vi "RF Rec Rx Streaming (Host).vi"() -> ()   [LabVIEW 2018]
doc: "This template is for the Simple NI-USRP Streaming design, a design that shows the basics of streaming data to and from an NI USRP-294x/295x device. Refer to the block diagram for more information about how to use this template."
uses:
  <vilib>/userdefined/Silver/nirio_resource_slv.ctl
  SubVIs/RF Rec Start Trigger.ctl
  <vilib>/Utility/error.llb/DialogType.ctl
panel:
  in  "config tab":enum32{"Rx Configuration"}(tab)
  in  "rx config":T2={"rf enable 0"=TRUE, "rf config 0"={"antenna"="RX2", "frequency"=2000000000.0, "lo frequency"=-1.0, "level"=0.0}, "rf enable 1"=TRUE, "rf config 1"={"antenna"="RX2", "frequency"=2000000000.0, "lo frequency"=-1.0, "level"=0.0}, "transfer mode"=enum."Finite", "sample rate"=10000000.0, "number of samples"=8192, "start trigger"=enum."Immediate"} {"sample rate" format="%#.3pS/s"; "rf config 1"."level" format="%#_gdBm"; "rf config 1"."lo frequency" format="%#.3pHz"; "rf config 1"."frequency" format="%#.3pHz"; "rf config 0"."level" format="%#_gdBm"; "rf config 0"."lo frequency" format="%#.3pHz"; "rf config 0"."frequency" format="%#.3pHz"}
  out "acquiring":bool caption="Acquiring"
  in  "USRP RIO device":T3="RIO0" caption="USRP RIO Device"
  in  "reference frequency source":string(combo)="Internal" caption="Reference Frequency Source"
  in  "indicator tab":T4(tab)
  out "power spectrum":cluster{"f0":dbl, "df":dbl, "magnitude":dbl[]}[](graph) caption="Power Spectrum"
  out "power level":dbl[][](graph) caption="Power Level"
  out "iq data":waveform(dbl)[](graph) caption="I & Q Data"
  out "rx.coerced config":T5 caption="Rx" {"coerced sample rates" format="%#.3pS/s"; "coerced levels" format="%#.3gdBm"; "coerced lo frequencies" format="%#.3pHz"; "coerced frequencies" format="%#.3pHz"}
  in  "rx.stop":bool
  # "This template is for the Simple NI-USRP Streaming design, a design that shows the basics of streaming data on a USRP RIO device. See the block diagram for more information on how to use this template."
  # "Simple Rx Streaming"
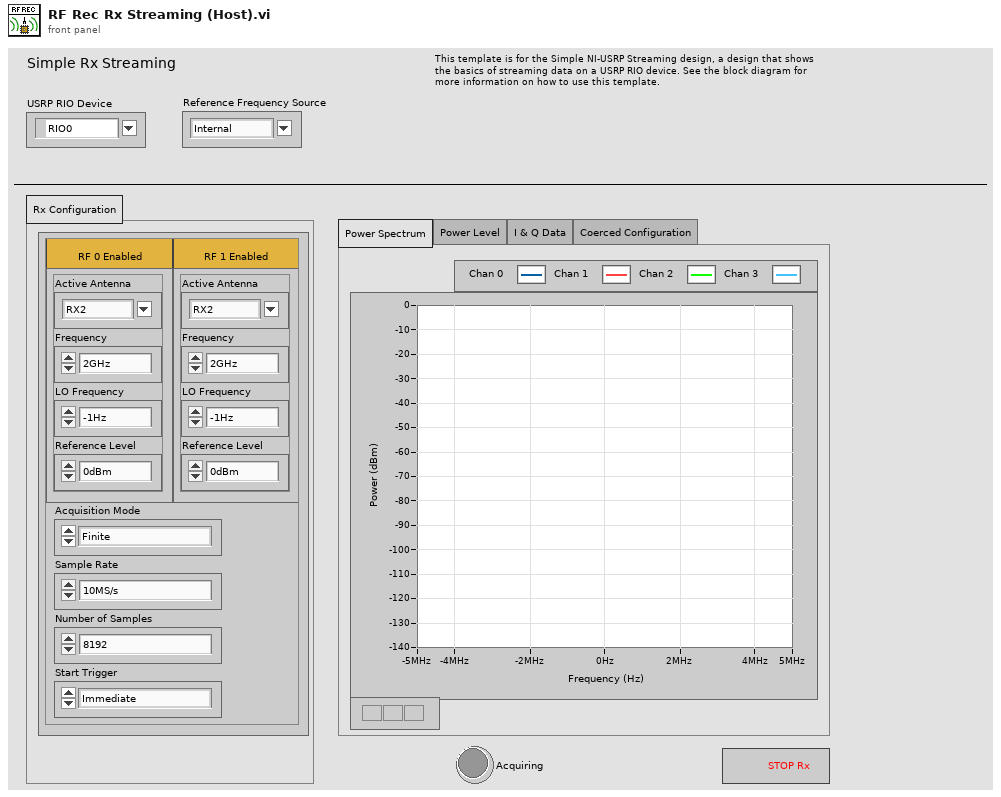
[diagram p1: front panel]
types:
  T1 = typedef "RF Rec Start Trigger.ctl" = enum8{"Software", "Digital Edge", "Rx Start Trigger", "Tx Start Trigger", "Immediate", "Future Time Event"}
  T2 = cluster{"rf enable 0":bool, "rf config 0":cluster{"antenna":string, "frequency":dbl, "lo frequency":dbl, "level":dbl}, "rf enable 1":bool, "rf config 1":cluster{"antenna":string, "frequency":dbl, "lo frequency":dbl, "level":dbl}, "transfer mode":enum16{"Finite", "Continuous"}, "sample rate":dbl, "number of samples":u32, "start trigger":T1}
  T3 = typedef "nirio_resource_slv.ctl" = tag
  T4 = enum32{"Power Spectrum", "Power Level", "I & Q Data", "Coerced Configuration"}
  T5 = cluster{"coerced frequencies":dbl[], "coerced lo frequencies":dbl[], "coerced levels":dbl[], "coerced sample rates":dbl[]}
  T6 = typedef "DialogType.ctl" = u16
  T7 = typedef "RF Rec Rx Channels.ctl" = cluster{"rx config":cluster{"channel configuration":cluster{"channel enable":bool, "channel configuration":cluster{"antenna":string, "frequency":dbl, "lo frequency":dbl, "level":dbl}}[], "transfer mode":enum16{"Finite", "Continuous"}, "sample rate":dbl, "number of samples":u32, "start trigger":T1}, "reference frequency source":string, "rx.data sink":enum16{"SFP Port 0", "SFP Port 1", "Host"}, "rx.enabled channels":string[], "vertical range":dbl[], "rx.coerced configurations":cluster{"coerced frequencies":dbl[], "coerced lo frequencies":dbl[], "coerced levels":dbl[], "coerced sample rates":dbl[]}}
  T8 = typedef "niUsrpRio Config v1 Host.lvlib/niUsrpRio Session.ctl" = cluster{"FPGA Interface":refnum<k20>, "RIO Interface Number":u32, "Data Clock Rate":u32, "FPGA Data Clock Rate":u32, "Global Settings Register Bus":T9, "Radio 0 Settings Register Bus":T9, "Radio 1 Settings Register Bus":T9, "Radio Settings Bus Semaphore":T10, "DB Queues":T11[], "Characterization Data Valid?":bool, "EEPROM Header":T12, "Device Data Header":T13, "EEPROM Characterization Header":T14, "Characterization Data":T15[], "FPGA Current Version":u32, "FPGA Oldest Compatible Version":u32, "Fixed Logic Current Version":u32, "Fixed Logic Oldest Compatible Version":u32, "FPGA Radio Settings Bus Current Version":u32, "FPGA Radio Settings Bus Oldest Compatible Version":u32, "FPGA Board Config Current Version":u32, "FPGA Board Config Oldest Compatible Version":u32, "Daughterboard Clock Rate":u32, "daughterboard configuration session handles":u64[]}
  T9 = typedef "niInstr Register Bus v0 Host.lvlib/Register Bus Session.ctl" = refnum<queue>
  T10 = typedef "Semaphore RefNum" = refnum<k1>
  T11 = typedef "niUsrpRio Config v1 Host.lvlib/DB Queue Reference.ctl" = refnum<queue>
  T12 = typedef "niUsrpRio Config v1 Host.lvlib/EEPROM Header.ctl" = cluster{"Checksum":u32, "Product Code":u16, "Hardware Current Version":u16, "Hardware Oldest Compatible Version":u16, "EEPROM Map Current Version":u16, "EEPROM Map Oldest Compatible Version":u16, "User Password":string, "Pointer to Factory Header":u32, "Pointer to User Header":u32, "Recommended Interval":u16, "Number of Reserved Bytes":i32, "Number of Daughterboards":u8, "Daughterboard IDs":u16[], "Daughterboard Serial Numbers":string[]}
  T13 = typedef "niUsrpRio Config v1 Host.lvlib/EEPROM Device Data Header.ctl" = cluster{"Checksum":u32, "Number of Channels":u8, "Number of Gain Settings":u16[], "Pointer to Characterization Data":u32[], "Number of Reserved Bytes":i32, "Number of Frequencies":u16[]}
  T14 = typedef "niUsrpRio Config v1 Host.lvlib/EEPROM Characterization Header.ctl" = cluster{"Checksum":u32, "Date":timestamp, "Temperature":sgl, "Misc. Info":string, "Pointer to Device Data Header":u32, "Number of Reserved Bytes":i32}
  T15 = typedef "niUsrpRio Config v1 Host.lvlib/Characterization Data.ctl" = cluster{"Gains[dB]":dbl[], "Frequencies [Hz]":dbl[], "IQ Imbalance Table":T16[], "Measured Gains[dB]":dbl[][]}
  T16 = typedef "niUsrpRio Config v1 Host.lvlib/IQ Imbalance.ctl" = cluster{"Gain Imbalance [linear]":dbl, "Phase Imbalance [radians]":dbl, "Offset":cdb}
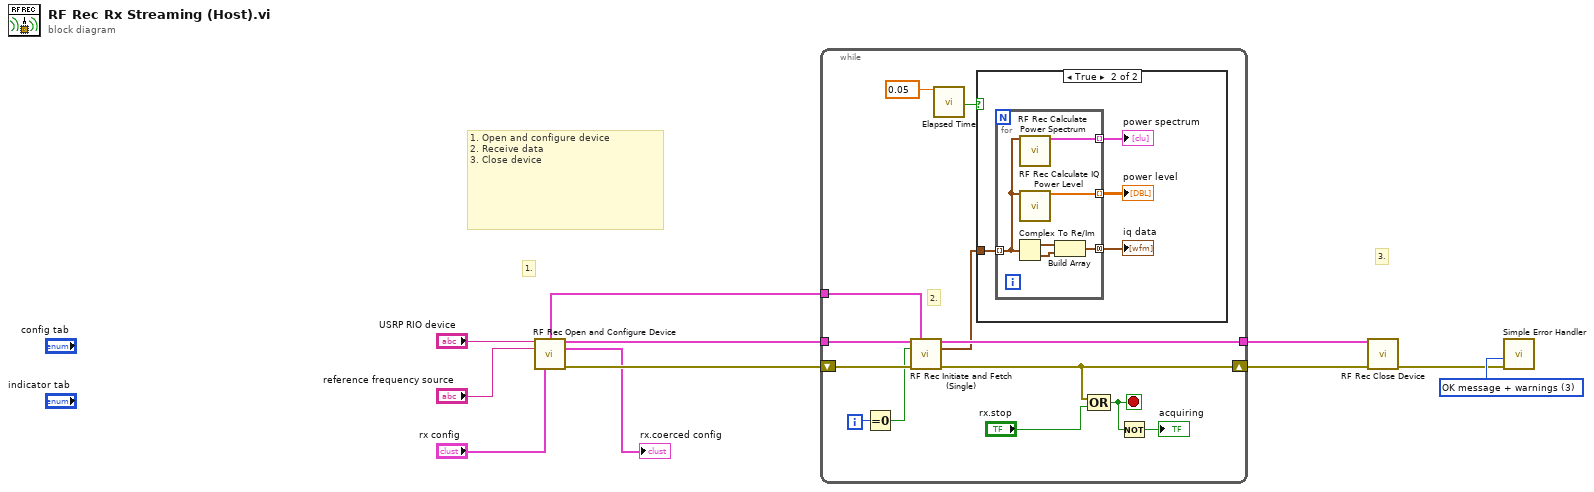
[diagram p0: block diagram]
diagram:
  w10 = T6 3 items=["no dialog", "OK message", "continue or stop message", "OK message + warnings", "continue/stop + warnings"] ("type of dialog (OK msg:1)")
  # "3."
  # "1. Open and configure device\n2. Receive data\n3. Close device"
  # "1."
  n1 = call "RF Rec Open and Configure Device.vi"("USRP RIO Device"="USRP RIO device", "reference frequency source"="reference frequency source", "rx config"="rx config") -> ("rx channels"=w8:T7, "niUsrpRio Session (out)"=w1:T8, "rx.coerced configurations"=→"rx.coerced config":T5, "error out"=w11:errorcluster)  [unwired: 6 in, 3 out]
  n2 = while {
    tunnel: w1 -> [w22]
    tunnel: [w19] -> w3
    tunnel: w8 -> [w16]
    shift-right: [w20] -> w4
    shift-left: w11 -> [w23]
    i -> [w21]
    stop <- w17 stop-if-true
    # "2."
    # "Acquire and Fetch a waveform"
    n3 = Equal To 0?(x=w21) -> (x = 0?=w12:bool)
    n4 = call "RF Rec Initiate and Fetch (Single).vi"("niUsrpRio Session"=w22, "rx channels"=w16, "first iteration"=w12, "error in"=w23) -> ("niUsrpRio Session (out)"=w19:T8, "complex baseband data"=w13:waveform(cdb)[], "error out"=w20:errorcluster)  [unwired: 9 in]
    n5 = call "Elapsed Time"("Time Target (s)"=0.05 ("retrigger delay")) -> ("Time has Elapsed"=w15:bool)  [unwired: 11 in, 7 out]
    n6 = case shown="True" w15 {
      tunnel: w13 -> [_ w28]
      frame False {
      }
      frame True {
        n7 = for {
          tunnel: [w32] -> w27 mode=concatenating
          tunnel: [w31] -> w26 mode=indexing
          tunnel: [w30] -> w25 mode=indexing
          tunnel: w28 -> [w29] mode=indexing
          n8 = Complex To Re/Im(x + iy=w29) -> (x=w34:waveform(dbl), y=w33:waveform(dbl))
          n9 = call "RF Rec Calculate Power Spectrum.vi"("waveform"=w29) -> ("power spectrum (dBm)"=w30:cluster{"f0":dbl, "df":dbl, "magnitude":dbl[]})  [unwired: 14 in]
          n10 = call "RF Rec Calculate IQ Power Level.vi"("iq data"=w29) -> ("power level (dBm)"=w31:dbl[])  [unwired: 14 in]
          n11 = Build Array(w34, w33) -> (w32:waveform(dbl)[])
        }
        "power level" <- w26
        "power spectrum" <- w25
        "iq data" <- w27
      }
    }
    n12 = Compound Arithmetic op=OR(w20, "rx.stop") -> (w17:bool)
    n13 = Not(x=w17) -> (.not. x?=→"acquiring":bool)
  }
  n14 = call "RF Rec Close Device.vi"("niUsrpRio Session"=w3, "error in"=w4) -> ("error out"=w9:errorcluster)  [unwired: 13 in]
  n15 = call <vilib>:"Simple Error Handler.vi"("type of dialog (OK msg:1)"=w10, "error in (no error)"=w9) -> ()  [unwired: 3 in, 5 out]
